vi "Weather Station UI.vi"() -> ()   [LabVIEW 2019]
uses:
  Supporting Files/Weather Station States.ctl
  Supporting Files/Weather Data.ctl
  <vilib>/DAQmx/read.llb/DAQmx Read (Analog DBL 1Chan 1Samp).vi
  <vilib>/DAQmx/create/channels.llb/DAQmx Create Channel (AI-Temperature-Thermocouple).vi
  <vilib>/DAQmx/miscellaneous.llb/DAQmx Fill In Error Info.vi
panel:
  in  "Stop":bool
  out "Warning":string
  out "Temperature History":dbl(graph)
  in  "Lower Limit":dbl=20.0
  in  "Upper Limit":dbl=30.0
  in  "Thermocouple Channel":tag="PCI-6221/ai0"
  # "Temperature Ranges (deg C)"
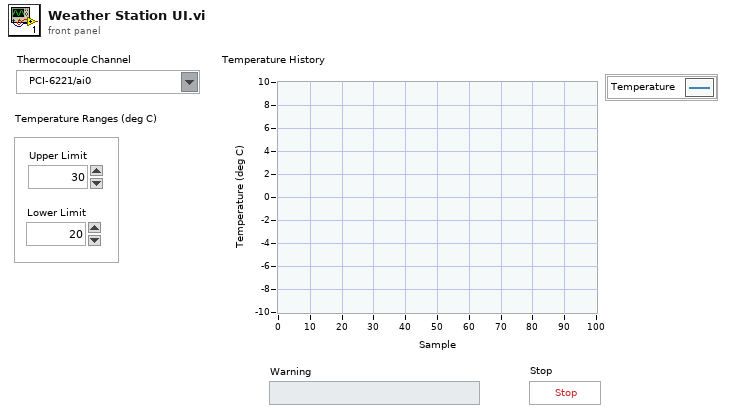
[diagram p1: front panel]
types:
  T1 = typedef "Weather Data.ctl" = cluster{"Current Temperature":dbl, "Max Temperature":dbl, "Min Temperature":dbl, "Warning?":bool, "Warning Text":string}
  T2 = enum16{"open", "replace", "create", "open or create", "replace or create", "replace or create with confirmation"}
  T3 = typedef "Weather Station States.ctl" = enum16{"Acquire", "Analyze", "Log", "Check Time"}
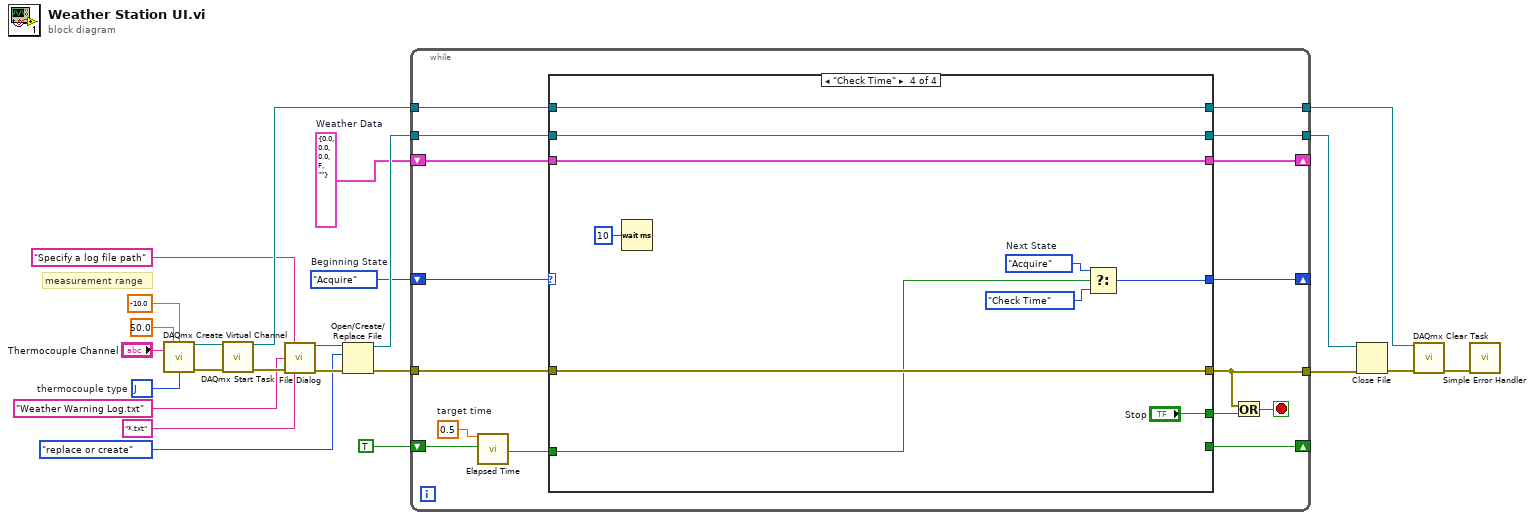
[diagram p0: block diagram]
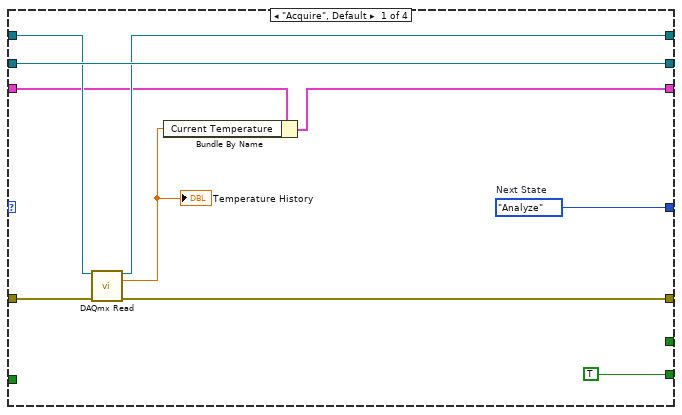
[diagram p2: hidden frame]
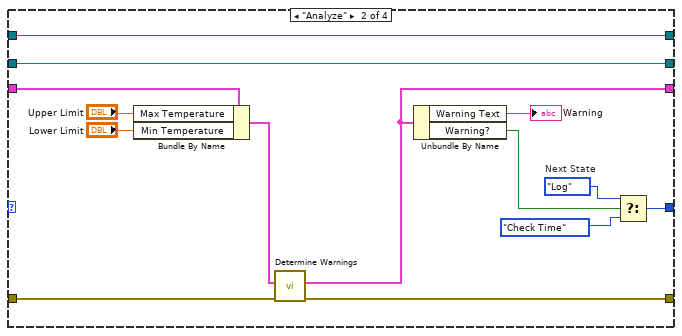
[diagram p3: hidden frame]
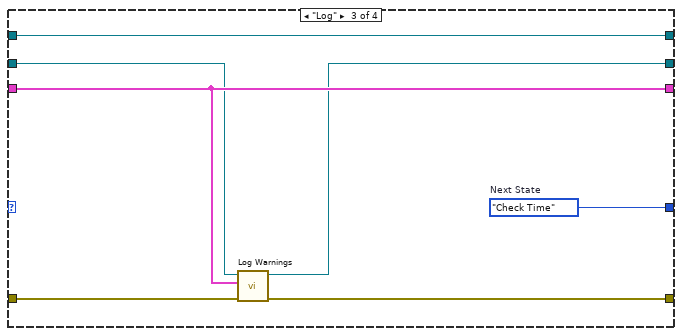
[diagram p4: hidden frame]
diagram:
  w1 = T1 {"Current Temperature"=0.0, "Max Temperature"=0.0, "Min Temperature"=0.0, "Warning?"=FALSE, "Warning Text"=""}  # Weather Data
  w7 = Weather_Station_States."Acquire"  # Beginning State
  w22 = 10072 items=["J"=10072, "K"=10073, "N"=10077, "R"=10082, "S"=10085, "T"=10086, "B"=10047, "E"=10055]  # thermocouple type
  # "measurement range"
  n1 = call-poly <vilib>:"DAQmx Create Virtual Channel.vi"("maximum value"=50.0, "minimum value"=-10.0, "physical channels"="Thermocouple Channel", "thermocouple type"=w22) -> ("task out"=w21:refnum<k21>, "error out"=w20:errorcluster)  [unwired: 10 in]
  n2 = call <vilib>:"DAQmx Start Task.vi"("task/channels in"=w21, "error in"=w20) -> ("task out"=w16:refnum<k21>, "error out"=w11:errorcluster)  [unwired: 12 in]
  n3 = call "File Dialog"("prompt"="Specify a log file path", "default name"="Weather Warning Log.txt", "error in"=w11, "pattern (all files)"="*.txt") -> ("selected path"=w18:path, "error out"=w19:errorcluster)  [unwired: 8 in, 2 out]
  n4 = Open/Create/Replace File(file path (use dialog)=w18, error in=w19, operation (0:open)=T2."replace or create") -> (refnum out=w17:refnum<file>, error out=w15:errorcluster)  [unwired: 3 in, 1 out]
  n5 = while {
    tunnel: w17 -> [w38]
    tunnel: w16 -> [w39]
    tunnel: w15 -> [w35]
    shift-right: [w28] -> _
    shift-left: TRUE -> [w26]
    shift-right: [w33] -> _
    shift-left: w1 -> [w36]
    shift-right: [w32] -> _
    shift-left: w7 -> [w37]
    tunnel: [w34] -> w5
    tunnel: [w29] -> w4
    tunnel: [w31] -> w6
    stop <- w30 stop-if-true
    w40 = 0.5  # target time
    n6 = call "Elapsed Time"("Time Target (s)"=w40, "Reset"=w26) -> ("Time has Elapsed"=w27:bool)  [unwired: 10 in, 7 out]
    n7 = case shown="\"Check Time\"" w37 {
      tunnel: w39 -> [w47 w57 w71 w80]
      tunnel: w38 -> [w50 w56 w67 w79]
      tunnel: w36 -> [w45 w64 w68 w78]
      tunnel: w35 -> [w49 w63 w70 w77]
      tunnel: [w44 w60 w68 w78] -> w33
      tunnel: [w50 w56 w66 w79] -> w31
      tunnel: [w48 w62 w69 w77] -> w29
      tunnel: [w46 w57 w71 w80] -> w34
      tunnel: [w41 w59 w65 w75] -> w32
      tunnel: [TRUE _ _ _] -> w28
      tunnel: w27 -> [_ _ _ w76]
      tunnel: [_ _ _ "Stop"] -> w25
      frame "Acquire", Default {
        w41 = Weather_Station_States."Analyze"  # Next State
        n8 = call-poly <vilib>:"DAQmx Read.vi"("task/channels in"=w47, "error in"=w49) -> ("task out"=w46:refnum<k21>, "data"=w42:dbl, "error out"=w48:errorcluster)  [unwired: 11 in]
        "Temperature History" <- w42
        n9 = Bundle By Name(cluster=w45, "Current Temperature"=w42) -> (w44:T1)
      }
      frame "Analyze" {
        w52 = Weather_Station_States."Log"  # Next State
        n10 = Bundle By Name(cluster=w64, "Max Temperature"="Upper Limit", "Min Temperature"="Lower Limit") -> (w61:T1)
        n11 = call "Determine Warnings.vi"("Error In"=w63, "Weather Data In"=w61) -> ("Error Out"=w62:errorcluster, "Weather Data Out"=w60:T1)  [unwired: 8 in]
        n12 = Unbundle By Name(w60) -> ("Warning Text"=→"Warning":string, "Warning?"=w58:bool)
        n13 = Select(t=w52, s=w58, f=Weather_Station_States."Check Time") -> (s? t:f=w59:T3)
      }
      frame "Log" {
        w65 = Weather_Station_States."Check Time"  # Next State
        n14 = call "Log Warnings.vi"("Error In"=w70, "Weather Data In"=w68, "file ref in"=w67) -> ("Error Out"=w69:errorcluster, "file ref out"=w66:refnum<file>)  [unwired: 7 in]
      }
      frame "Check Time" {
        w73 = Weather_Station_States."Acquire"  # Next State
        n15 = Wait (ms)(milliseconds to wait=u32 10) -> ()  [unwired: 1 out]
        n16 = Select(t=w73, s=w76, f=Weather_Station_States."Check Time") -> (s? t:f=w75:T3)
      }
    }
    n17 = Or(x=w29, y=w25) -> (x .or. y?=w30:bool)
  }
  n18 = Close File(refnum=w6, error in=w4) -> (error out=w13:errorcluster)  [unwired: 1 out]
  n19 = call <vilib>:"DAQmx Clear Task.vi"("task in"=w5, "error in"=w13) -> ("error out"=w12:errorcluster)  [unwired: 13 in]
  n20 = call <vilib>:"Simple Error Handler.vi"("error in (no error)"=w12) -> ()  [unwired: 4 in, 5 out]
